vi "DriveExecute.vi"(8 "error in (no error)":errorcluster) -> (0 "error out":errorcluster)   [LabVIEW 2023]
doc: "Execute for Drie\n\nClosed control loop for drive\n\ninput: \n error in (cluster)\n\noutput:\n error out (cluster)"
uses:
  <vilib>/Rock Robotics/WPI/ThirdParty/JAS_Junk/TrajLib/LinearFilter_ResetToValue.vi
  <vilib>/Rock Robotics/WPI/ThirdParty/JAS_Junk/TrajLib/LinearFilter_Calculate.vi
  DriveGlobal.vi
  <vilib>/Rock Robotics/WPI/ThirdParty/JAS_Junk/TrajLib/LinearFilter_MovingAverage.vi
  <vilib>/Rock Robotics/WPI/ThirdParty/JAS_Junk/TrajLib/LinearFilter_LowPassBW1.vi
  <vilib>/Rock Robotics/WPI/ThirdParty/JAS_Junk/TrajLib/LinearFilter_LowPassBW2.vi
  <vilib>/Rock Robotics/WPI/ThirdParty/JAS_Junk/TrajLib/LinearFilter_HighPassBW1.vi
  <vilib>/Rock Robotics/WPI/ThirdParty/JAS_Junk/TrajLib/LinearFilter_HighPassBW2.vi
  <vilib>/Rock Robotics/WPI/ThirdParty/JAS_Junk/TrajLib/Trajectory_Library.lvlib
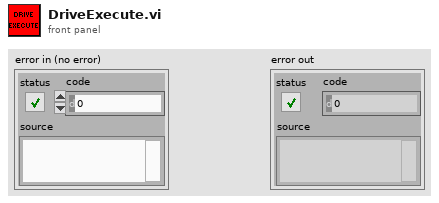
[diagram p1: front panel]
types:
  T1 = enum16{"Moving Average", "Low Pass 1st Order Butterworth", "Low Pass 2nd Order Butterworth", "High Pass 1st Order Butterworth", "High Pass 2nd Order Butterworth"}
  T2 = typedef "Trajectory_Library.lvlib/CHASSIS_SPEEDS.ctl" = cluster{"vX":dbl, "vY":dbl, "vOmega":dbl}
  T3 = typedef "ADIS16470 Device Reference.ctl" = cluster{"DevStatus":errorcluster, "Hardware Config":T4, "Calibration Complete":refnum<notifier>, "Status Reference":refnum<data-value>, "Data Reference":refnum<data-value>, "Sychronous Process VI":T8, "Cmd FIFO":refnum<k33>, "Source":T9, "Data FIFO":refnum<k33>, "Calibration Time (ms)":u32, "Data Reference":refnum<data-value>}
  T4 = typedef "ADIS16470 Hardware Configuration.ctl" = cluster{"SPI Clock Rate (Hz)":dbl, "IMU SPI Mode (3)":T5, "IMU Reset Pin":T6, "IMU SPI Bus":T7, "IMU Data Ready Pin":T6, "Stall Config":cluster{"Pow2BytesPerRead":u8, "StallTicks":u16, "CsToSclkTicks":u8}}
  T5 = typedef "WPI_SPIMode.ctl" = enum16{"Mode 0 (Clk Idle Low,Sample on Leading)", "Mode 1 (Clk Idle Low,Sample on Trailing)", "Mode 2 (Clk Idle High,Sample on Leading)", "Mode 3 (Clk Idle High,Sample on Trailing)"}
  T6 = typedef "FPGA_DIOChannel.ctl" = enum8{"DIO 0", "DIO 1", "DIO 2", "DIO 3", "DIO 4", "DIO 5", "DIO 6", "DIO 7", "DIO 8", "DIO 9", "DIO MXP 0", "DIO MXP 1", "DIO MXP 2", "DIO MXP 3", "DIO MXP 4", "DIO MXP 5", "DIO MXP 6", "DIO MXP 7", "DIO MXP 8", "DIO MXP 9", "DIO MXP 10", "DIO MXP 11", "DIO MXP 12", "DIO MXP 13", "DIO MXP 14", "DIO MXP 15", "SPI Port CS1", "SPI Port CS2", "SPI Port CS3", "SPI Port MISO", "SPI Port MOSI", "Invalid"}
  T7 = typedef "spi_bus.ctl" = enum16{"SPI On-Board, CS0", "SPI On-Board, CS1", "SPI On-Board, CS2", "SPI On-Board, CS3", "SPI MXP", "Invalid"}
  T8 = typedef "ADIS16470 Process.ctl" = refnum<vi>
  T9 = typedef "FPGA_CounterEncoderSourceConvertionLVSourceType.ctl" = cluster{"DevStatus":errorcluster, "AnalogTriggerMode?":bool, "DigitalMode":cluster{"DIO Channel":T10}, "AnalogTriggerMode":cluster{"AnalogTriggerIndex":T11, "OutputType":T12}}
  T10 = typedef "FPGA_DIODigitalSourceChannel.ctl" = enum8{"DIO 0", "DIO 1", "DIO 2", "DIO 3", "DIO 4", "DIO 5", "DIO 6", "DIO 7", "DIO 8", "DIO 9", "DIO MXP 0", "DIO MXP 1", "DIO MXP 2", "DIO MXP 3", "DIO MXP 4", "DIO MXP 5", "DIO MXP 6", "DIO MXP 7", "DIO MXP 8", "DIO MXP 9", "DIO MXP 10", "DIO MXP 11", "DIO MXP 12", "DIO MXP 13", "DIO MXP 14", "DIO MXP 15", "SPI Port CS1", "SPI Port CS2", "SPI Port CS3", "SPI Port MISO", "SPI Port MOSI", "Disabled"}
  T11 = typedef "FPGA_AnalogTriggerIndex.ctl" = enum8{"Trig 0", "Trig 1", "Trig 2", "Trig 3", "Trig 4", "Trig 5", "Trig 6", "Trig 7", "Invalid"}
  T12 = typedef "FPGA_AnalogTriggerOutType.ctl" = enum16{"InWindow", "TriggerState", "Rising", "Falling"}
  T13 = typedef "Trajectory_Library.lvlib/SWERVE_DRIVE_KINEMATICS.ctl" = cluster{"NumModules":i32, "InverseKinematics":T14, "ForwardKinematics":T14, "Modules":T15[], "PrevCoR":T15, "SavedModuleStates":T16[]}
  T14 = typedef "NI_Matrix.lvlib/RealMatrix.ctl" = dbl[][]
  T15 = typedef "Trajectory_Library.lvlib/TRANSLATION2D.ctl" = cluster{"X":dbl, "Y":dbl}
  T16 = typedef "Trajectory_Library.lvlib/SWERVE_DRIVE_MODULE_STATE.ctl" = cluster{"Speed":dbl, "Angle":T17}
  T17 = typedef "Trajectory_Library.lvlib/ROTATION2D.ctl" = cluster{"VALUE":dbl, "COS":dbl, "SIN":dbl}
  T18 = typedef "ADIS16470 Status.ctl" = cluster{"Calibrated?":bool, "IMU Detected?":bool}
  T19 = typedef "Trajectory_Library.lvlib/SWERVE_DRIVE_MODULE_POSITION.ctl" = cluster{"Distance":dbl, "Angle":T17, "P":bool}
  T20 = typedef "ADIS16470 Data.ctl" = cluster{"XAngle":dbl, "YAngle":dbl, "ZAngle":dbl}
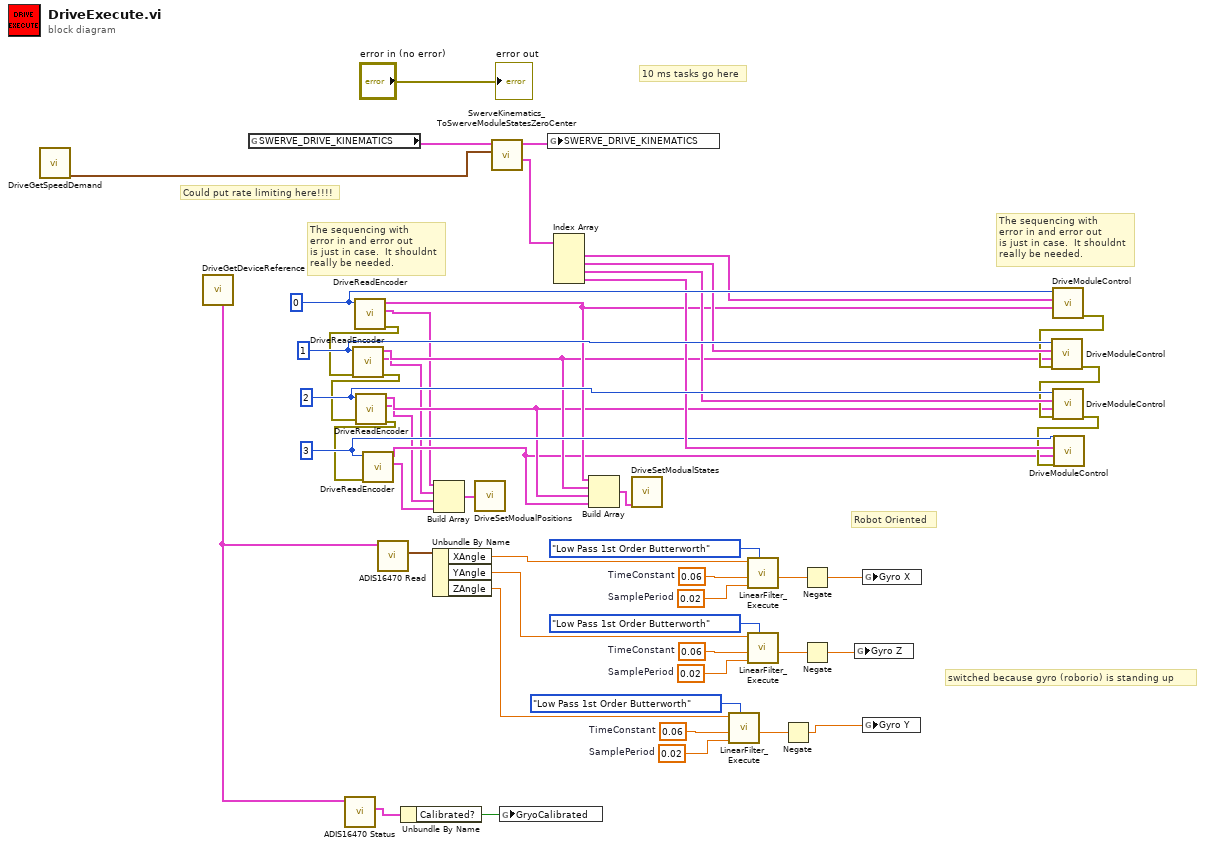
[diagram p0: block diagram]
diagram:
  w27 = 0 ("ModualNamePrefix")
  w26 = 1 ("ModualNamePrefix")
  w25 = 2 ("ModualNamePrefix")
  w19 = 3 ("ModualNamePrefix")
  w36 = 0.02  # SamplePeriod
  w35 = 0.06  # TimeConstant
  w41 = 0.02  # SamplePeriod
  w40 = 0.06  # TimeConstant
  w46 = 0.02  # SamplePeriod
  w45 = 0.06  # TimeConstant
  # "The sequencing with\nerror in and error out\nis just in case.  It shouldnt\nreally be needed."
  # "The sequencing with\nerror in and error out\nis just in case.  It shouldnt\nreally be needed."
  # "Could put rate limiting here!!!!"
  # "switched because gyro (roborio) is standing up"
  # "Robot Oriented"
  # "10 ms tasks go here"
  n1 = call "DriveGetSpeedDemand.vi"() -> ("ChassisSpeedDemand"=w29:T2)  [unwired: 8 in, 3 out]
  n2 = call "DriveGetDeviceReference.vi"() -> ("Gryo"=w47:T3)  [unwired: 11 in]
  n3 = global read "DriveGlobal.vi" "SWERVE_DRIVE_KINEMATICS"() -> (w30:T13)
  n4 = call <vilib>:"ADIS16470 Status.vi"("ADIS16470DevRef"=w47) -> ("ADIS16470 Status"=w49:T18)  [unwired: 8 in, 2 out]
  n5 = call "DriveReadEncoder.vi"("ModualNamePrefix"=w27) -> ("error out"=w3:errorcluster, "SWERVE_DRIVE_MODULE_POSITION"=w11:T19, "SWERVE_DRIVE_MODULE_STATE"=w15:T16)  [unwired: 8 in]
  n6 = call "DriveReadEncoder.vi"("error in"=w3, "ModualNamePrefix"=w26) -> ("error out"=w2:errorcluster, "SWERVE_DRIVE_MODULE_POSITION"=w10:T19, "SWERVE_DRIVE_MODULE_STATE"=w14:T16)  [unwired: 7 in]
  n7 = call "DriveReadEncoder.vi"("error in"=w2, "ModualNamePrefix"=w25) -> ("error out"=w1:errorcluster, "SWERVE_DRIVE_MODULE_POSITION"=w9:T19, "SWERVE_DRIVE_MODULE_STATE"=w13:T16)  [unwired: 7 in]
  n8 = call "DriveReadEncoder.vi"("error in"=w1, "ModualNamePrefix"=w19) -> ("SWERVE_DRIVE_MODULE_POSITION"=w8:T19, "SWERVE_DRIVE_MODULE_STATE"=w12:T16)  [unwired: 7 in, 1 out]
  n9 = call <vilib>:"ADIS16470 Read.vi"("ADIS16470DevRef"=w47) -> ("ADIS16470 Value"=w50:T20)  [unwired: 7 in, 3 out]
  n10 = Unbundle By Name(w49) -> ("Calibrated?"=w48:bool)
  n11 = Unbundle By Name(w50) -> ("XAngle"=w31:dbl, "YAngle"=w37:dbl, "ZAngle"=w43:dbl)
  n12 = Build Array(w11, w10, w9, w8) -> (w6:T19[])
  n13 = call "DriveSetModualPositions.vi"("Swerve_Drive_Modual_Position"=w6) -> ()  [unwired: 11 in]
  n14 = call <vilib>:"SwerveKinematics_ToSwerveModuleStatesZeroCenter.vi"("ChassisSpeeds"=w29, "in SWERVE_DRIVE_KINEMATICS"=w30) -> ("ModuleStates"=w24:T16[], "out SWERVE_DRIVE_KINEMATICS"=w28:T13)  [unwired: 8 in]
  n15 = global write "DriveGlobal.vi" "GryoCalibrated"(w48) -> ()
  n16 = global write "DriveGlobal.vi" "SWERVE_DRIVE_KINEMATICS"(w28) -> ()
  n17 = Index Array(array=w24) -> (element #1=w20:T16, element #2=w23:T16, element #3=w22:T16, element #4=w21:T16)  [unwired: 4 in]
  n18 = Build Array(w15, w14, w13, w12) -> (w7:T16[])
  n19 = call "DriveSetModualStates.vi"("Swerve__Drive_Modual_States"=w7) -> ()  [unwired: 11 in]
  n20 = call <vilib>:"LinearFilter_Execute.vi"("Filter Type"=T1."Low Pass 1st Order Butterworth", "SamplePeriod"=w46, "TimeConstant"=w45, "Input"=w43) -> ("Output"=w42:dbl)  [unwired: 6 in, 1 out]
  n21 = call <vilib>:"LinearFilter_Execute.vi"("Filter Type"=T1."Low Pass 1st Order Butterworth", "SamplePeriod"=w36, "TimeConstant"=w35, "Input"=w31) -> ("Output"=w33:dbl)  [unwired: 6 in, 1 out]
  n22 = call <vilib>:"LinearFilter_Execute.vi"("Filter Type"=T1."Low Pass 1st Order Butterworth", "SamplePeriod"=w41, "TimeConstant"=w40, "Input"=w37) -> ("Output"=w38:dbl)  [unwired: 6 in, 1 out]
  n23 = Negate(x=w42) -> (-x=w4:dbl)
  n24 = Negate(x=w33) -> (-x=w32:dbl)
  n25 = Negate(x=w38) -> (-x=w5:dbl)
  n26 = global write "DriveGlobal.vi" "Gyro Z"(w5) -> ()
  n27 = global write "DriveGlobal.vi" "Gyro X"(w32) -> ()
  n28 = global write "DriveGlobal.vi" "Gyro Y"(w4) -> ()
  n29 = call "DriveModuleControl.vi"("Actual State"=w15, "Desired State"=w20, "ModualNamePrefix"=w27) -> ("error out"=w18:errorcluster)  [unwired: 8 in]
  n30 = call "DriveModuleControl.vi"("error in"=w18, "Actual State"=w14, "Desired State"=w23, "ModualNamePrefix"=w26) -> ("error out"=w17:errorcluster)  [unwired: 7 in]
  n31 = call "DriveModuleControl.vi"("error in"=w17, "Actual State"=w13, "Desired State"=w22, "ModualNamePrefix"=w25) -> ("error out"=w16:errorcluster)  [unwired: 7 in]
  n32 = call "DriveModuleControl.vi"("error in"=w16, "Actual State"=w12, "Desired State"=w21, "ModualNamePrefix"=w19) -> ()  [unwired: 7 in, 1 out]
  "error out" <- "error in (no error)"
